vi "Enable Channel.vi"(7 "Simulation":T1, 8 "error in":errorcluster, 9 "String":string, 10 "Args":string[](array[string]), 11 "Ophir Pulsar in":refnum<class "Ophir Juno.lvclass">) -> (0 "error out":errorcluster, 2 "new commands":string, 3 "Ophir Pulsar out":refnum<class "Ophir Juno.lvclass">)   [LabVIEW 2020, in "Ophir Juno.lvclass"]
uses:
  Ophir Juno.lvclass
  OnOffTypeDef.ctl
  Enable_Disable Channel.ctl
  Ophir Juno.lvclass/Ophir Juno.ctl
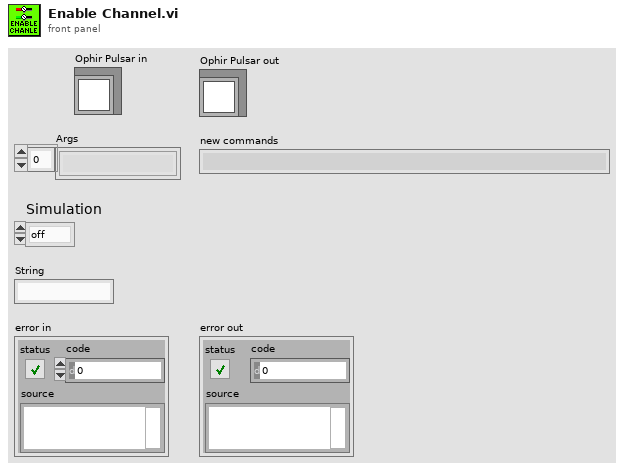
[diagram p1: front panel]
types:
  T1 = typedef "OnOffTypeDef.ctl" = enum16{"off", "on"}
  T2 = typedef "Ophir Juno.lvclass/Enable_Disable Channel.ctl" = enum16{"Enable", "Disable"}
  T3 = cluster{"Channel0":T2, "Channel1":T2, "Channel2":T2, "Channel3":T2}
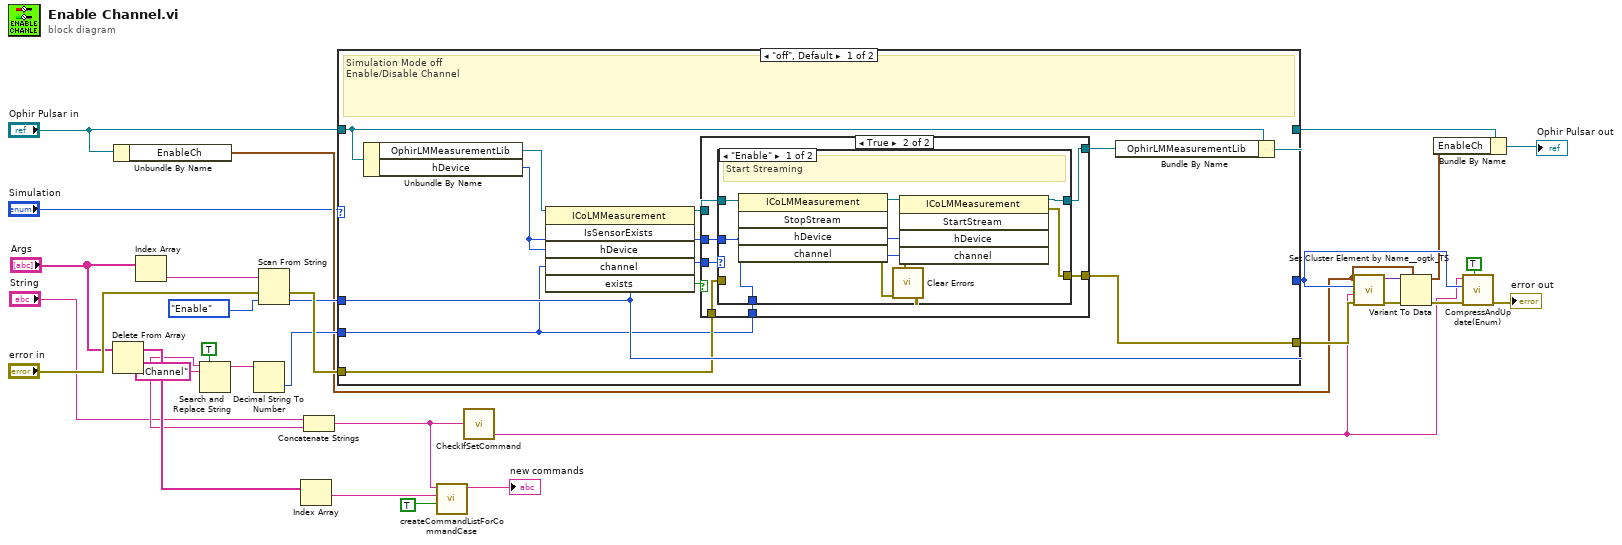
[diagram p0: block diagram]
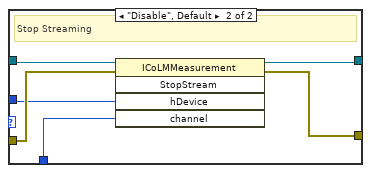
[diagram p3: hidden frame]
diagram:
  n1 = Delete From Array(array="Args") -> (deleted portion=w11:string, array with subset deleted=w17:string[])  [unwired: 2 in]
  n2 = Unbundle By Name("Ophir Pulsar in") -> ("EnableCh"=w13:T3)
  n3 = Index Array(array="Args") -> (element=w23:string)  [unwired: 1 in]
  n4 = Search and Replace String(replace all?=TRUE ("replace all? (F)"), input string=w11, search string=".Channel") -> (result string=w15:string)  [unwired: 5 in, 3 out]
  n5 = Decimal String To Number(string=w15) -> (number=w30:i32)  [unwired: 2 in, 1 out]
  n6 = Scan From String(input string=w23, error in="error in", default 1=Enable_Disable_Channel."Enable") -> (error out=w31:errorcluster, output 1=w24:T2)  [unwired: 2 in, 2 out]
  n7 = Index Array(array=w17) -> (element=w18:string)  [unwired: 1 in]
  n8 = Concatenate Strings("String", w11) -> (w16:string)
  n9 = case shown="\"off\", Default" "Simulation" {
    tunnel: w24 -> [w40 w68]
    tunnel: [w40 w68] -> w26
    tunnel: w31 -> [w39 w67]
    tunnel: [w38 w67] -> w27
    tunnel: "Ophir Pulsar in" -> [w42 w66]
    tunnel: [w41 w66] -> w20
    tunnel: w30 -> [w32 _]
    frame "off", Default {
      # "Simulation Mode off\nEnable/Disable Channel"
      n10 = Unbundle By Name(w42) -> ("OphirLMMeasurementLib"=w36:refnum<k7>, "hDevice"=w33:i32)
      n11 = invoke class="ICoLMMeasurement" method="IsSensorExists"(reference=w36, "hDevice"=w33, "channel"=w32) -> (reference out=w35:refnum<k7>, "exists"=w34:bool)  [unwired: 3 in, 4 out]
      n12 = case shown="True" w34 {
        tunnel: w40 -> [_ w51]
        tunnel: w33 -> [_ w50]
        tunnel: w32 -> [_ w49]
        tunnel: w39 -> [w43 w48]
        tunnel: [w43 w47] -> w38
        tunnel: [w44 w46] -> w37
        tunnel: w35 -> [w44 w45]
        frame False {
        }
        frame True {
          n13 = case shown="\"Enable\"" w51 {
            tunnel: w50 -> [w56 w63]
            tunnel: w49 -> [w57 w62]
            tunnel: w45 -> [w55 w65]
            tunnel: w48 -> [_ w64]
            tunnel: [w59 w61] -> w47
            tunnel: [w58 w60] -> w46
            frame "Enable" {
              # "Start Streaming"
              n14 = invoke class="ICoLMMeasurement" method="StopStream"(reference=w55, "hDevice"=w56, "channel"=w57) -> (reference out=w54:refnum<k7>, error out=w53:errorcluster)  [unwired: 2 in, 3 out]
              n15 = call "Clear Errors.vi"("error in (no error)"=w53) -> ("error out"=w52:errorcluster)  [unwired: 5 in, 1 out]
              n16 = invoke class="ICoLMMeasurement" method="StartStream"(reference=w54, error in=w52, "hDevice"=w56, "channel"=w57) -> (reference out=w58:refnum<k7>, error out=w59:errorcluster)  [unwired: 1 in, 3 out]
            }
            frame "Disable", Default {
              # "Stop Streaming"
              n17 = invoke class="ICoLMMeasurement" method="StopStream"(reference=w65, error in=w64, "hDevice"=w63, "channel"=w62) -> (reference out=w60:refnum<k7>, error out=w61:errorcluster)  [unwired: 1 in, 3 out]
            }
          }
        }
      }
      n18 = Bundle By Name(cluster=w42, "OphirLMMeasurementLib"=w37) -> (w41:refnum<class "Ophir Juno.lvclass">)
    }
    frame "on" {
      # "Simulation Mode on"
    }
  }
  n19 = call "createCommandListForCommandCase.vi"("immediate Check (only once)"=TRUE, "setvalue"=w18, "command"=w16) -> ("new commands"=→"new commands":string)  [unwired: 8 in]
  n20 = call "CheckIfSetCommand.vi"("Command"=w16) -> ("variable"=w10:string)  [unwired: 2 out]
  n21 = call "Set Cluster Element by Name__ogtk_TS.vi"("error in (no error)"=w27, "Element Name (\"\": New Element Data Name)"=w10, "New Element Value"=w26, "Cluster"=w13) -> ("error out"=w28:errorcluster, "VCluster out"=w14:variant)  [unwired: 5 in, 1 out]
  n22 = Variant To Data(error in=w28, type=w13, Variant=w14) -> (data=w12:T3, error out=w29:errorcluster)
  n23 = Bundle By Name(cluster=w20, "EnableCh"=w12) -> (→"Ophir Pulsar out":refnum<class "Ophir Juno.lvclass">)
  n24 = call "CompressAndUpdate(Enum).vi"("force CVT update (false)"=TRUE, "error in"=w29, "enum variant"=w26, "command or variable name"=w10) -> ("error out"=→"error out":errorcluster)  [unwired: 7 in]
